vi "VI-FILE-DACS MASTER.vi"() -> ()   [LabVIEW 2013]
panel:
  out "DRAWING ROOM OA":bool
  out "DINING ROOM OA":bool
  out "LIBRARY OA":bool
  out "CHAMBER OA":bool
  out "DRAWING ROOM LED":bool
  out "DINING ROOM LED":bool
  out "LIBRARY LED":bool
  out "CHAMBER LED":bool
  out "LIBRARY LT F VIS OO\nREMOTE triigger 4":bool
  out "DRAWING ROOM LT S VIS OO\nREMOTE triigger 3":bool
  out "DINING ROOM LT S VIS OO":bool
  out "CHAMBER LT F VIS OO":bool
  out "REMOTE CONFIRMATION\nREMOTE triigger 2":bool
  out "DINING ROOM LT S OO":bool
  out "DRAWING ROOM LT S OO":bool
  out "LIBRARY LT OO\nLOCAL trigger":bool
  out "CHAMBER LT OO\nLOCAL trigger":bool
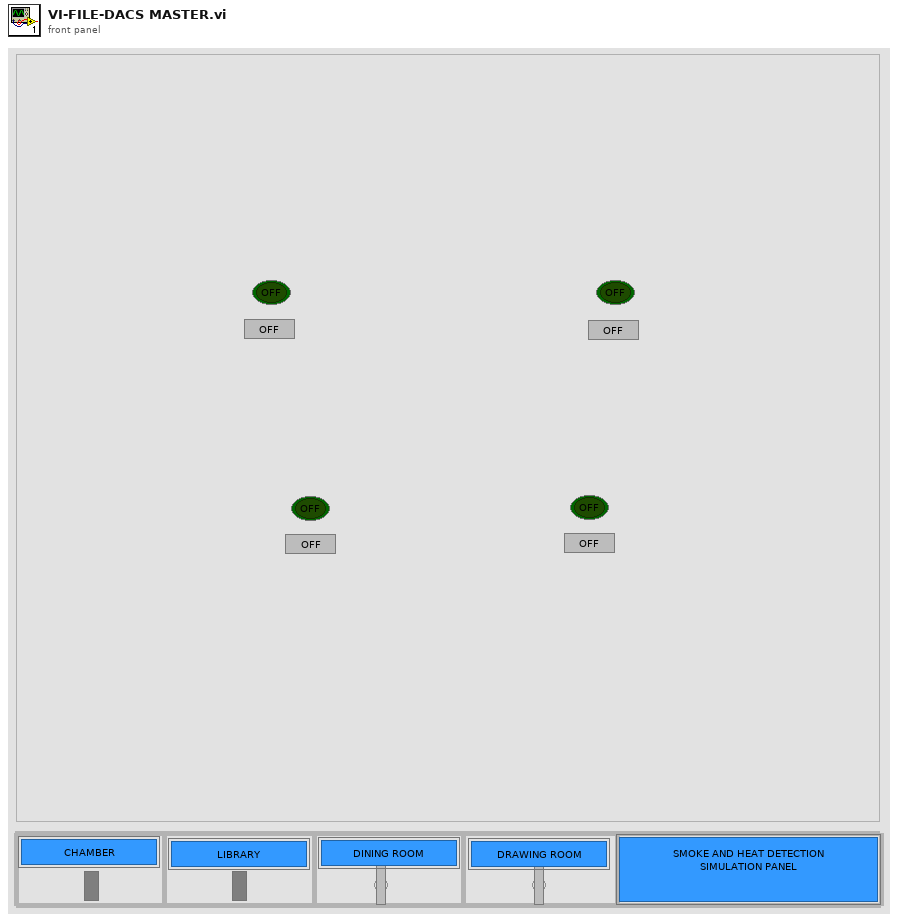
[diagram p1: front panel]
types:
  T1 = cluster{"data[0]":bool, "data[1]":bool, "data[2]":bool, "data[3]":bool, "data[4]":bool, "data[5]":bool, "data[6]":bool, "data[7]":bool, "data[8]":bool}
  T2 = cluster{"CHAMBER LED":bool, "LIBRARY LED":bool, "DINING ROOM LED":bool, "DRAWING ROOM LED":bool}
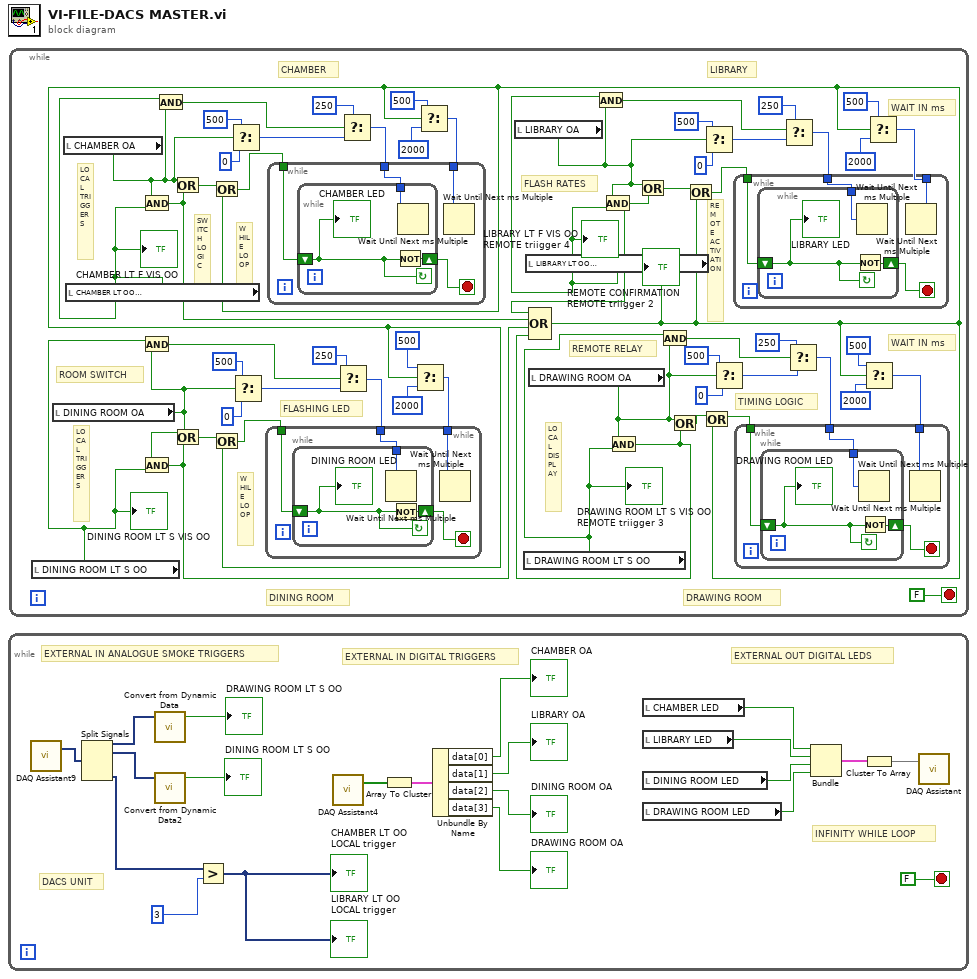
[diagram p0: block diagram]
diagram:
  n1 = while {
    stop <- FALSE stop-if-true
    # "INFINITY WHILE LOOP"
    # "DACS UNIT"
    # "EXTERNAL OUT DIGITAL LEDS"
    # "EXTERNAL IN DIGITAL TRIGGERS"
    # "EXTERNAL IN ANALOGUE SMOKE TRIGGERS"
    n2 = call "DAQ Assistant9"() -> ("data"=w20:dynamicdata)  [unwired: 17 in, 2 out]
    n3 = Split Signals(w20) -> (w19:dynamicdata, w18:dynamicdata, w3:dynamicdata)  [unwired: 5 in, 2 out]
    n4 = call "Convert from Dynamic Data"("Dynamic Data Type"=w19) -> ("Scalar"=→"DRAWING ROOM LT S OO":bool)  [unwired: 3 in]
    n5 = call "Convert from Dynamic Data2"("Dynamic Data Type"=w18) -> ("Scalar"=→"DINING ROOM LT S OO":bool)  [unwired: 3 in]
    n6 = Greater?(x=w3, y=3) -> (0:→"CHAMBER LT OO\nLOCAL trigger" →"LIBRARY LT OO\nLOCAL trigger":dynamicdata)
    n7 = call "DAQ Assistant4"() -> ("data"=w17:bool[])  [unwired: 17 in, 2 out]
    n8 = Array To Cluster(array=w17) -> (cluster=w16:T1)
    n9 = Unbundle By Name(w16) -> ("data[0]"=→"CHAMBER OA":bool, "data[1]"=→"LIBRARY OA":bool, "data[2]"=→"DINING ROOM OA":bool, "data[3]"=→"DRAWING ROOM OA":bool)
    n10 = local read "CHAMBER LED"() -> (w11:bool)
    n11 = local read "LIBRARY LED"() -> (w10:bool)
    n12 = local read "DINING ROOM LED"() -> (w9:bool)
    n13 = local read "DRAWING ROOM LED"() -> (w8:bool)
    n14 = Bundle("CHAMBER LED"=w11, "LIBRARY LED"=w10, "DINING ROOM LED"=w9, "DRAWING ROOM LED"=w8) -> (w7:T2)  [unwired: 1 in]
    n15 = Cluster To Array(cluster=w7) -> (array=w6:bool[])
    n16 = call "DAQ Assistant"("data"=w6) -> ()  [unwired: 17 in, 2 out]
  }
  n17 = while {
    stop <- FALSE stop-if-true
    # "FLASH RATES"
    # "WHILE LOOP"
    # "WHILE LOOP"
    # "ROOM SWITCH"
    # "WAIT IN ms"
    # "LOCAL DISPLAY"
    # "LOCAL TRIGGERS"
    # "REMOTE RELAY"
    # "WAIT IN ms"
    # "TIMING LOGIC"
    # "SWITCH LOGIC"
    # "LOCAL TRIGGERS"
    # "REMOTE ACTIVATION"
    # "FLASHING LED"
    # "DRAWING ROOM"
    # "DINING ROOM"
    # "LIBRARY"
    # "CHAMBER"
    n18 = local read "DINING ROOM LT S OO"() -> (w29:bool)
    "DINING ROOM LT S VIS OO" <- w29
    n19 = local read "DINING ROOM OA"() -> (w26:bool)
    n20 = local read "CHAMBER OA"() -> (w27:bool)
    n21 = local read "CHAMBER LT OO\nLOCAL trigger"() -> (w23:bool)
    "CHAMBER LT F VIS OO" <- w23
    n22 = And(x=w27, y=w23) -> (x .and. y?=w79:bool)
    n23 = And(x=w29, y=w26) -> (x .and. y?=w33:bool)
    n24 = And(x=w26, y=w29) -> (x .and. y?=w78:bool)
    n25 = And(x=w23, y=w27) -> (x .and. y?=w35:bool)
    n26 = Or(x=w27, y=w79) -> (x .or. y?=w74:bool)
    n27 = Or(x=w26, y=w78) -> (x .or. y?=w73:bool)
    n28 = Select(t=u32 500, s=w27, f=u32 0) -> (s? t:f=w65:u32)
    n29 = Select(t=u32 500 ("millisecond timer value"), s=w26, f=u32 0) -> (s? t:f=w51:u32)
    n30 = Select(t=u32 250, s=w33, f=w51) -> (s? t:f=w53:u32)
    n31 = Select(t=u32 250, s=w35, f=w65) -> (s? t:f=w37:u32)
    n32 = local read "LIBRARY OA"() -> (w25:bool)
    n33 = local read "DRAWING ROOM LT S OO"() -> (w30:bool)
    "DRAWING ROOM LT S VIS OO\nREMOTE triigger 3" <- w30
    n34 = local read "LIBRARY LT OO\nLOCAL trigger"() -> (w22:bool)
    "LIBRARY LT F VIS OO\nREMOTE triigger 4" <- w22
    n35 = local read "DRAWING ROOM OA"() -> (w24:bool)
    n36 = And(x=w22, y=w25) -> (x .and. y?=w34:bool)
    n37 = And(x=w25, y=w22) -> (x .and. y?=w38:bool)
    n38 = And(x=w24, y=w30) -> (x .and. y?=w77:bool)
    n39 = Compound Arithmetic op=OR ("REMOTE trigger")(w38, w79, w78, w77) -> (w31:bool)
    "REMOTE CONFIRMATION\nREMOTE triigger 2" <- w31
    n40 = Or(x=w74, y=w31) -> (x .or. y?=w72:bool)
    n41 = Or(x=w73, y=w31) -> (x .or. y?=w69:bool)
    n42 = Select(t=u32 500, s=w31, f=u32 2000 ("millisecond timer value")) -> (s? t:f=w55:u32)
    n43 = while {
      tunnel: w69 -> [w82]
      tunnel: w55 -> [w81]
      tunnel: w53 -> [w80]
      stop <- w83 stop-if-true
      n44 = while {
        shift-right: [w86] -> w83
        shift-left: w82 -> [w84]
        tunnel: w80 -> [w85]
        stop <- w84 continue-if-true
        n45 = Wait Until Next ms Multiple(millisecond multiple=w85) -> ()  [unwired: 1 out]
        n46 = Not(x=w84) -> (.not. x?=w86:bool)
        "DINING ROOM LED" <- w84
      }
      n47 = Wait Until Next ms Multiple(millisecond multiple=w81) -> ()  [unwired: 1 out]
    }
    n48 = Select(t=u32 500, s=w31, f=u32 2000 ("millisecond timer value")) -> (s? t:f=w39:u32)
    n49 = while {
      tunnel: w72 -> [w103]
      tunnel: w39 -> [w102]
      tunnel: w37 -> [w101]
      stop <- w104 stop-if-true
      n50 = while {
        shift-right: [w107] -> w104
        shift-left: w103 -> [w105]
        tunnel: w101 -> [w106]
        stop <- w105 continue-if-true
        n51 = Not(x=w105) -> (.not. x?=w107:bool)
        n52 = Wait Until Next ms Multiple(millisecond multiple=w106) -> ()  [unwired: 1 out]
        "CHAMBER LED" <- w105
      }
      n53 = Wait Until Next ms Multiple(millisecond multiple=w102) -> ()  [unwired: 1 out]
    }
    n54 = Or(x=w25, y=w38) -> (x .or. y?=w76:bool)
    n55 = And(x=w30, y=w24) -> (x .and. y?=w32:bool)
    n56 = Or(x=w24, y=w77) -> (x .or. y?=w75:bool)
    n57 = Or(x=w76, y=w31) -> (x .or. y?=w71:bool)
    n58 = Or(x=w75, y=w31) -> (x .or. y?=w70:bool)
    n59 = Select(t=u32 500, s=w25, f=u32 0) -> (s? t:f=w59:u32)
    n60 = Select(t=u32 500, s=w24, f=u32 0) -> (s? t:f=w46:u32)
    n61 = Select(t=u32 250 ("millisecond timer value"), s=w34, f=w59) -> (s? t:f=w58:u32)
    n62 = Select(t=u32 250, s=w32, f=w46) -> (s? t:f=w42:u32)
    n63 = Select(t=u32 500, s=w31, f=u32 2000 ("millisecond timer value")) -> (s? t:f=w41:u32)
    n64 = while {
      tunnel: w70 -> [w89]
      tunnel: w41 -> [w88]
      tunnel: w42 -> [w87]
      stop <- w90 stop-if-true
      n65 = while {
        shift-right: [w93] -> w90
        shift-left: w89 -> [w91]
        tunnel: w87 -> [w92]
        stop <- w91 continue-if-true
        n66 = Wait Until Next ms Multiple(millisecond multiple=w92) -> ()  [unwired: 1 out]
        n67 = Not(x=w91) -> (.not. x?=w93:bool)
        "DRAWING ROOM LED" <- w91
      }
      n68 = Wait Until Next ms Multiple(millisecond multiple=w88) -> ()  [unwired: 1 out]
    }
    n69 = Select(t=u32 500, s=w31, f=u32 2000 ("millisecond timer value")) -> (s? t:f=w40:u32)
    n70 = while {
      tunnel: w71 -> [w96]
      tunnel: w40 -> [w95]
      tunnel: w58 -> [w94]
      stop <- w97 stop-if-true
      n71 = while {
        shift-right: [w100] -> w97
        shift-left: w96 -> [w98]
        tunnel: w94 -> [w99]
        stop <- w98 continue-if-true
        n72 = Not(x=w98) -> (.not. x?=w100:bool)
        n73 = Wait Until Next ms Multiple(millisecond multiple=w99) -> ()  [unwired: 1 out]
        "LIBRARY LED" <- w98
      }
      n74 = Wait Until Next ms Multiple(millisecond multiple=w95) -> ()  [unwired: 1 out]
    }
  }
